vi "Initialize Data Reader.vi"(8 "error in (no error)":errorcluster, 11 "Phasor Data Concentrator in":refnum<class "Phasor Data Concentrator.lvclass">) -> (0 "error out":errorcluster, 3 "Phasor Data Concentrator out":refnum<class "Phasor Data Concentrator.lvclass">)   [LabVIEW 2012]
uses:
  PMU Recorder Light.lvlib
  Phasor Data Concentrator.lvclass
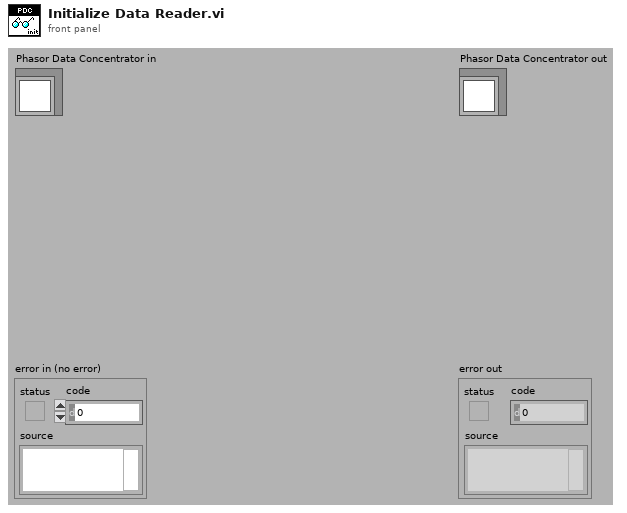
[diagram p1: front panel]
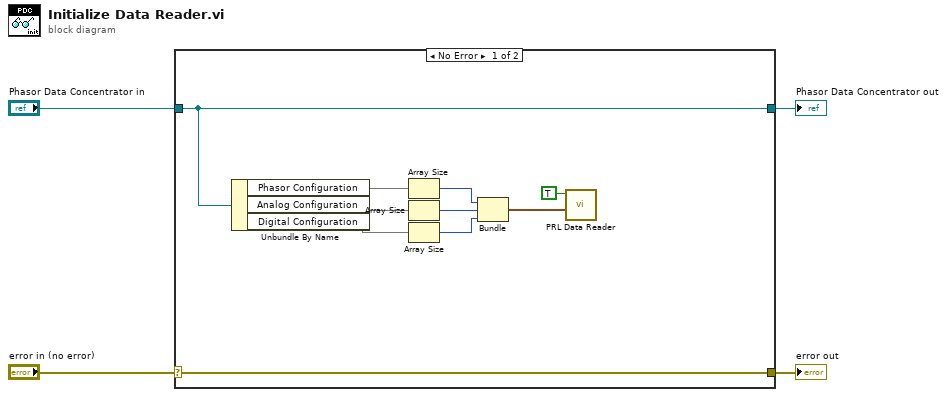
[diagram p0: block diagram]
diagram:
  n1 = case shown="No Error" "error in (no error)" {
    selector: "error in (no error)" -> [w14 w16]
    tunnel: [w14 w16] -> w3
    tunnel: [w13 w15] -> w1
    tunnel: "Phasor Data Concentrator in" -> [w13 w15]
    frame No Error {
      n2 = Unbundle By Name(w13) -> ("Phasor Configuration"=w12, "Analog Configuration"=w11, "Digital Configuration"=w10)
      n3 = Array Size(array=w12) -> (size(s)=w9:i32)
      n4 = Array Size(array=w11) -> (size(s)=w8:i32)
      n5 = Array Size(array=w10) -> (size(s)=w7:i32)
      n6 = Bundle(w9, w8, w7) -> (w6:cluster{i32, i32, i32})  [unwired: 1 in]
      n7 = call "PRL Data Reader.vi"("Initialize Data"=w6, "Initialize"=TRUE ("Initialize Buffers?")) -> ()  [unwired: 3 in, 7 out]
    }
    frame Error {
    }
  }
  "error out" <- w3
  "Phasor Data Concentrator out" <- w1
